vi "Get column name.vi"(8 "error in (no error)":errorcluster, 11 "Column Interface in":refnum<class "Column Interface.lvclass">) -> (0 "error out":errorcluster, 2 "Name":string, 3 "Column Interface out":refnum<class "Column Interface.lvclass">)   [LabVIEW 2020, in "Column Interfaces.lvlib" / "Column Interface.lvclass"]
uses:
  Column Interface.lvclass
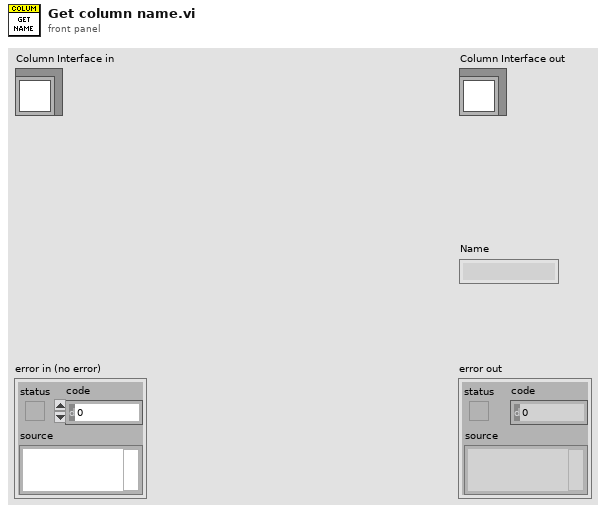
[diagram p1: front panel]
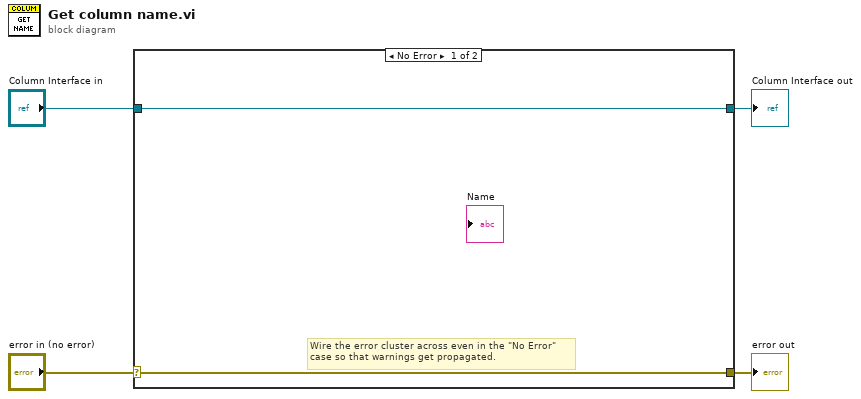
[diagram p0: block diagram]
diagram:
  n1 = case shown="No Error" "error in (no error)" {
    selector: "error in (no error)" -> [w5 w8]
    tunnel: [w5 w8] -> w3
    tunnel: [w6 w7] -> w1
    tunnel: "Column Interface in" -> [w6 w7]
    frame No Error {
      # "Wire the error cluster across even in the \"No Error\"\ncase so that warnings get propagated."
    }
    frame Error {
    }
  }
  "error out" <- w3
  "Column Interface out" <- w1
